vi "RP Read Temperature.vi"(8 "Error In":errorcluster, 11 "connection ID":refnum<k5>) -> (0 "error out":errorcluster, 2 "Thermometer":dbl(slide)=48.847186279148 scale=0.0..100.0, 3 "connection ID out":refnum<k5>)   [LabVIEW 2015]
uses:
  RP Command.ctl
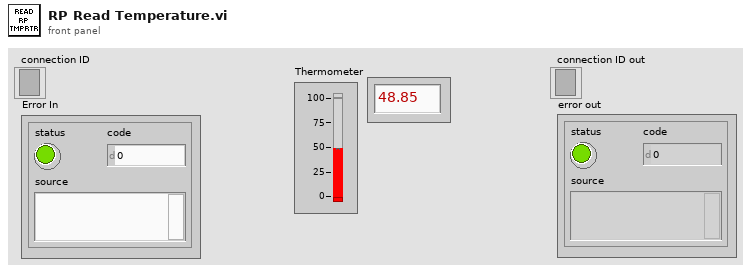
[diagram p1: front panel]
types:
  T1 = enum16{"big-endian, network order", "native, host order", "little-endian"}
  T2 = typedef "RP Command.ctl" = enum16{"Set frequency", "Arm and get data", "Stop server", "Get status", "Get temperature", "Set decimation", "Arm", "Software trigger", "Get whole buffer", "Get chunk", "System call", "Get config", "Set config"}
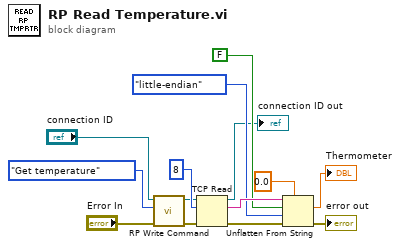
[diagram p0: block diagram]
diagram:
  n1 = call "RP Write Command.vi"("Error In"="Error In", "Command number"=RP_Command."Get temperature", "connection ID"="connection ID") -> ("Error Out"=w7:errorcluster, "connection ID out"=w6:refnum<k5>)  [unwired: 6 in, 1 out]
  n2 = TCP Read(connection ID=w6, bytes to read=8, error in (no error)=w7) -> (connection ID out=→"connection ID out":refnum<k5>, data out=w13:string, error out=w11:errorcluster)  [unwired: 2 in]
  n3 = Unflatten From String(type=0.0, binary string=w13, data includes array or string size? (T)=FALSE, byte order (0:big-endian, network order)=T1."little-endian", error in (no error)=w11) -> (value=→"Thermometer":dbl, error out=→"error out":errorcluster)  [unwired: 1 out]
